vi "CheckHandle.vi"(8 "error in (no error)":errorcluster, 10 "Array":T1(array[cluster]), 11 "Handle In":string) -> (0 "error out":errorcluster, 1 "instrument handle out":refnum<k15>, 2 "Handle Connected?":bool, 3 "Handle Out":string)   [LabVIEW 2018, in "AcPwrPlugins.lvlib" / "ChromaPowerSupply.lvclass"]
uses:
  ChromaPowerSupply.lvclass
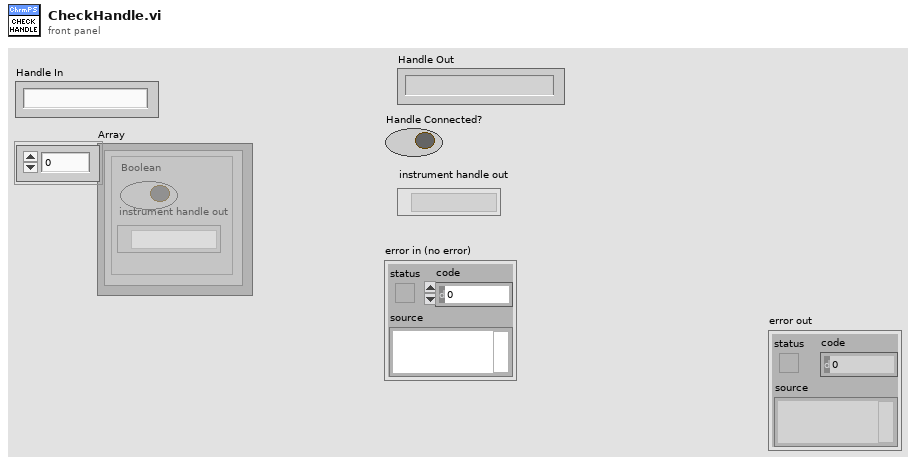
[diagram p1: front panel]
types:
  T1 = cluster{"Boolean":bool, "instrument handle out":refnum<k15>}[]
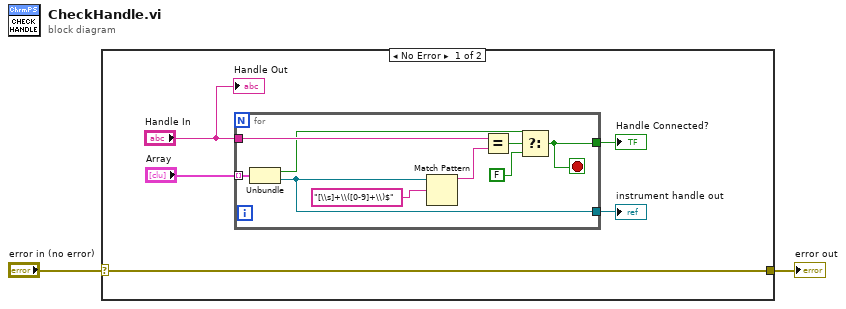
[diagram p0: block diagram]
diagram:
  n1 = case shown="No Error" "error in (no error)" {
    selector: "error in (no error)" -> [w5 w17]
    tunnel: [w5 w17] -> w1
    frame No Error {
      n2 = for {
        tunnel: "Handle In" -> [w16]
        tunnel: [w14] -> w6
        tunnel: "Array" -> [w10] mode=indexing
        tunnel: [w8] -> w3
        stop <- w14 stop-if-true
        n3 = Unbundle(w10) -> ("Boolean"=w9:bool, "instrument handle out"=w8:refnum<k15>)
        n4 = Match Pattern(string=w8, regular expression="[\\s]+\\([0-9]+\\)$") -> (before substring=w12:string)  [unwired: 1 in, 3 out]
        n5 = Equal?(x=w16, y=w12) -> (x = y?=w15:bool)
        n6 = Select(t=w9, s=w15, f=FALSE) -> (s? t:f=w14:bool)
      }
      "Handle Connected?" <- w6
      "instrument handle out" <- w3
      "Handle Out" <- "Handle In"
    }
    frame Error {
    }
  }
  "error out" <- w1
